vi "MGI Set Listbox Scrollbar.vi"(10 "Error In":errorcluster, 11 "Listbox Reference In":refnum<vi>) -> (2 "Error Out":errorcluster, 3 "Listbox Reference Out":refnum<vi>)   [LabVIEW 2020]
doc: "Show or hide the specified listbox's vertical scrollbar based on the listbox contents. This VI will also set the scrollbar position as necessary to ensure that some of the listbox's contents is displayed.\n\nAuthored by Shawn Walpole\nsupport@mooregoodideas.com\nwww.mooregoodideas.com\n\nCopyright (c) 2010, Moore Good Ideas, Inc.\n\nAll rights reserved.\n\nRedistribution and use in source and binary forms, with or without modification, are permitted provided that the following conditions are met:\n\n * Redistributions of source code must retain the above copyright notice, this list of conditions and the following disclaimer.\n * Redistributions in binary form must reproduce the above copyright notice, this list of conditions and the following disclaimer in the documentation and/or other materials provided with the distribution.\n * Neither the name of Moore Good Ideas, Inc. nor the names of its contributors may be used to endorse or promote products derived from this software without specific prior written permission.\n\nTHIS SOFTWARE IS PROVIDED BY THE COPYRIGHT HOLDERS AND CONTRIBUTORS \"AS IS\" AND ANY EXPRESS OR IMPLIED WARRANTIES, INCLUDING, BUT NOT LIMITED TO, THE IMPLIED WARRANTIES OF MERCHANTABILITY AND FITNESS FOR A PARTICULAR PURPOSE ARE DISCLAIMED. IN NO EVENT SHALL THE COPYRIGHT OWNER OR CONTRIBUTORS BE LIABLE FOR ANY DIRECT, INDIRECT, INCIDENTAL, SPECIAL, EXEMPLARY, OR CONSEQUENTIAL DAMAGES (INCLUDING, BUT NOT LIMITED TO, PROCUREMENT OF SUBSTITUTE GOODS OR SERVICES; LOSS OF USE, DATA, OR PROFITS; OR BUSINESS INTERRUPTION) HOWEVER CAUSED AND ON ANY THEORY OF LIABILITY, WHETHER IN CONTRACT, STRICT LIABILITY, OR TORT (INCLUDING NEGLIGENCE OR OTHERWISE) ARISING IN ANY WAY OUT OF THE USE OF THIS SOFTWARE, EVEN IF ADVISED OF THE POSSIBILITY OF SUCH DAMAGE."
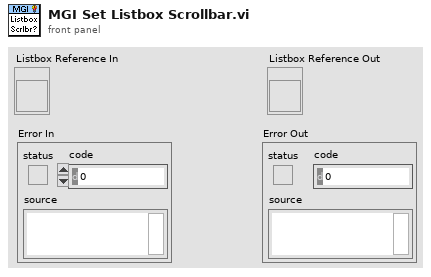
[diagram p1: front panel]
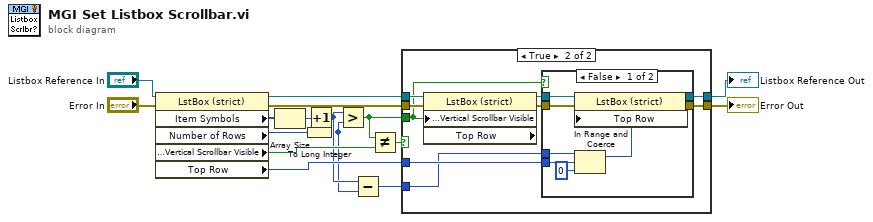
[diagram p0: block diagram]
diagram:
  n1 = property class="LstBox (strict)"(reference="Listbox Reference In", error in="Error In") -> (reference out=w16:refnum<vi>, error out=w7:errorcluster, "Item Symbols"=w14:i32[], "Number of Rows"=w3:u32, "Visible Items:Vertical Scrollbar Visible"=w12:bool, "Top Row"=w5:i32)
  n2 = Array Size(array=w14) -> (size(s)=w13:i32)
  n3 = To Long Integer(number=w3) -> (32bit integer=w1:i32)
  n4 = Increment(x=w13) -> (x+1=w4:i32)
  n5 = Greater?(x=w4, y=w1) -> (0:w11:bool)
  n6 = Subtract(x=w4, y=w1) -> (x-y=w2:i32)
  n7 = Not Equal?(x=w11, y=w12) -> (x != y?=w10:bool)
  n8 = case shown="True" w10 {
    tunnel: w16 -> [w18 w27]
    tunnel: w11 -> [_ w21]
    tunnel: [w18 w23] -> w9
    tunnel: w7 -> [w17 w26]
    tunnel: [w17 w22] -> w6
    tunnel: w5 -> [_ w20]
    tunnel: w2 -> [_ w19]
    frame False {
    }
    frame True {
      n9 = property class="LstBox (strict)" props=["Visible Items:Vertical Scrollbar Visible", "Top Row"](reference=w27, error in=w26, "Visible Items:Vertical Scrollbar Visible"=w21) -> (reference out=w25:refnum<vi>, error out=w24:errorcluster)  [unwired: 1 out]
      n10 = case shown="False" w21 {
        tunnel: w25 -> [w35 w37]
        tunnel: w24 -> [w34 w36]
        tunnel: [w33 w37] -> w23
        tunnel: [w32 w36] -> w22
        tunnel: w20 -> [w31 _]
        tunnel: w19 -> [w28 _]
        frame False {
          n11 = In Range and Coerce(upper limit=w28, x=w31, lower limit=0) -> (coerced(x)=w30:i32)  [unwired: 1 out]
          n12 = property class="LstBox (strict)"(reference=w35, error in=w34, "Top Row"=w30) -> (reference out=w33:refnum<vi>, error out=w32:errorcluster)
        }
        frame True {
        }
      }
    }
  }
  "Listbox Reference Out" <- w9
  "Error Out" <- w6
